vi "parse byte array.vi"(11 "byte array":u8[](array[numeric])) -> (3 "elements":T1[](array[typedef]))   [LabVIEW 2013, in "protocol buffers encoder.lvlib"]
uses:
  protocol buffers encoder.lvlib
  semiparse.ctl
  wire type.ctl
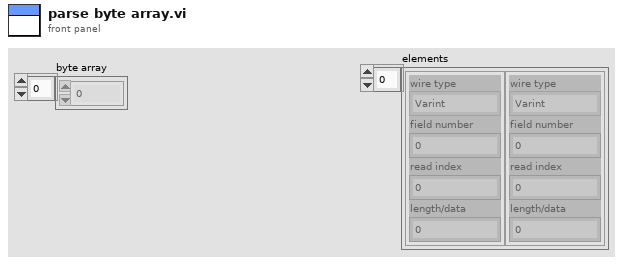
[diagram p1: front panel]
types:
  T1 = typedef "protocol buffers encoder.lvlib/semiparse.ctl" = cluster{"wire type":T2, "field number":u64, "read index":i32, "length/data":u64}
  T2 = typedef "protocol buffers encoder.lvlib/wire type.ctl" = enum8{"Varint", "64 bit", "Length Delimited", "Start Group", "End Group", "32 bit"}
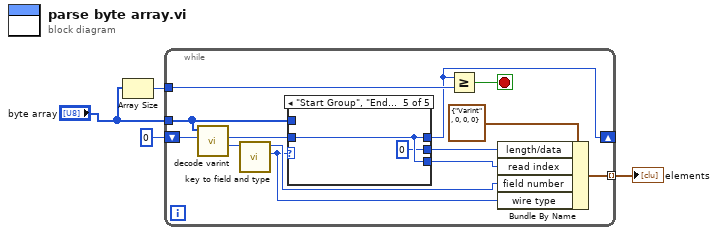
[diagram p0: block diagram]
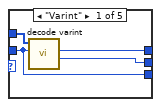
[diagram p2: hidden frame]
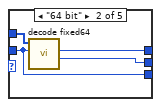
[diagram p3: hidden frame]
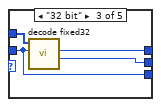
[diagram p4: hidden frame]
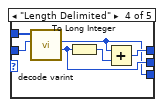
[diagram p5: hidden frame]
diagram:
  n1 = Array Size(array="byte array") -> (size(s)=w3:i32)
  n2 = while {
    tunnel: "byte array" -> [w9]
    shift-right: [w8] -> _
    shift-left: 0 -> [w17]
    tunnel: w3 -> [w15]
    tunnel: [w11] -> w2 mode=indexing
    stop <- w16 stop-if-true
    n3 = call "decode varint.vi"("read index in"=w17, "byte array in"=w9) -> ("value"=w14:u64, "read index out"=w7:i32)  [unwired: 8 in]
    n4 = call "key to field and type.vi"("key"=w14) -> ("wire type"=w10:T2, "field number"=w12:u64)  [unwired: 9 in]
    n5 = case shown="\"Start Group\", \"End Group\"" w10 {
      tunnel: w9 -> [w21 w25 w29 w35 _]
      tunnel: [w20 w23 w27 w34 w37] -> w8
      tunnel: w7 -> [w19 w24 w28 w31 w37]
      tunnel: [w18 w22 w26 w33 u64 0 ("u64")] -> w6
      tunnel: [w19 w24 w28 w30 w37] -> w5
      frame "Varint" {
        n6 = call "decode varint.vi"("read index in"=w19, "byte array in"=w21) -> ("value"=w18:u64, "read index out"=w20:i32)  [unwired: 8 in]
      }
      frame "64 bit" {
        n7 = call "decode fixed64.vi"("read index in"=w24, "byte array in"=w25) -> ("u64"=w22:u64, "read index out"=w23:i32)  [unwired: 8 in]
      }
      frame "32 bit" {
        n8 = call "decode fixed32.vi"("read index in"=w28, "byte array in"=w29) -> ("u32"=w26:u32, "read index out"=w27:i32)  [unwired: 8 in]
      }
      frame "Length Delimited" {
        n9 = call "decode varint.vi"("read index in"=w31, "byte array in"=w35) -> ("value"=w33:u64, "read index out"=w30:i32)  [unwired: 8 in]
        n10 = To Long Integer(number=w33) -> (32bit integer=w32:i32)
        n11 = Add(x=w30, y=w32) -> (x+y=w34:i32)
      }
      frame "Start Group", "End Group" {
      }
    }
    n12 = Greater Or Equal?(x=w8, y=w15) -> (x >= y?=w16:bool)
    n13 = Bundle By Name(cluster=T1 {"wire type"=enum."Varint", "field number"=0, "read index"=0, "length/data"=0} ("semiparse"), "length/data"=w6, "read index"=w5, "field number"=w12, "wire type"=w10) -> (w11:T1)
  }
  "elements" <- w2
